vi "Test for Progress Bar Popup.vi"() -> ()   [LabVIEW 2014]
panel:
  in  "Abort visible? (T)":bool=TRUE
  in  "mS delay per iteration":i32=100
  in  "Number of iterations":u32=47
  in  "Go":bool
  in  "Stop Button":bool
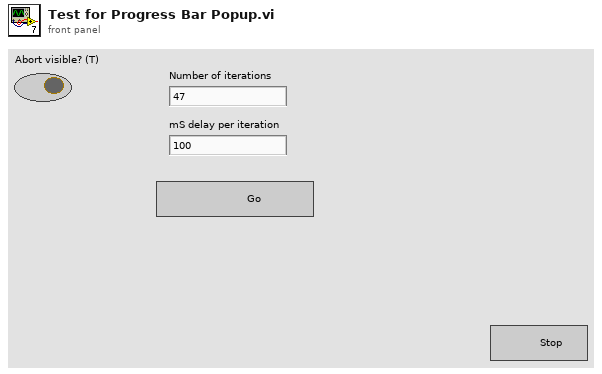
[diagram p1: front panel]
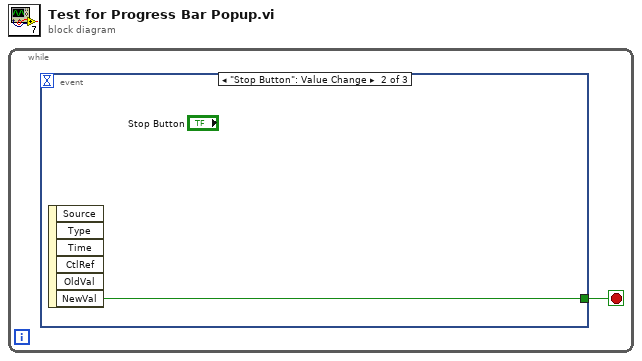
[diagram p0: block diagram]
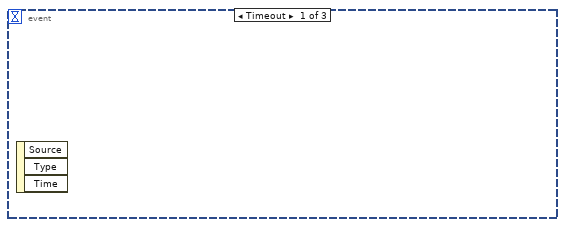
[diagram p2: hidden frame]
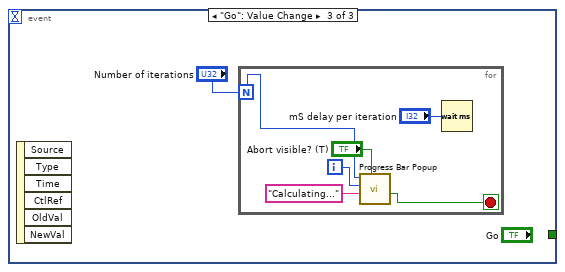
[diagram p3: hidden frame]
diagram:
  n1 = while {
    stop <- w1 stop-if-true
    n2 = event shown="[1] \"Stop Button\": Value Change" {
      selector: _ -> [_ _ _]
      dyn-events: _ -> [_ _ _]
      timeout: _ -> [_ _ _]
      tunnel: [_ w2 _] -> w1
      event Timeout {
        n3 = event-data() -> ()  [unwired: 1 in, 3 out]
      }
      event "Stop Button": Value Change {
        n4 = event-data() -> ("NewVal"=w2:bool)  [unwired: 1 in, 5 out]
      }
      event "Go": Value Change {
        n5 = event-data() -> ()  [unwired: 1 in, 6 out]
        n6 = for {
          N: "Number of iterations" -> [w8]
          i -> [w7]
          stop <- w5 stop-if-true
          n7 = call "Progress Bar Popup.vi"("Abort visible? (T)"="Abort visible? (T)", "Message (Please Wait...)"="Calculating...", "Current Iteration"=w7, "Total Iterations"=w8) -> ("Aborted"=w5:bool)  [unwired: 7 in]
          n8 = Wait (ms)(milliseconds to wait="mS delay per iteration") -> ()  [unwired: 1 out]
        }
      }
    }
  }
